vi "Set Error Line Format.vi"(8 "error in (no error)":errorcluster, 10 "Error Line Format":string, 11 "HSE_v2_Formatter in":refnum<class "HSE_v2_Formatter.lvclass">) -> (0 "error out":errorcluster, 3 "HSE_v2_Formatter out":refnum<class "HSE_v2_Formatter.lvclass">)   [LabVIEW 2016, in "hse-logger.lvlib" / "HSE_v2_Formatter.lvclass"]
uses:
  HSE_v2_Formatter.lvclass
  HSE_v2_Formatter.lvclass/HSE_v2_Formatter.ctl
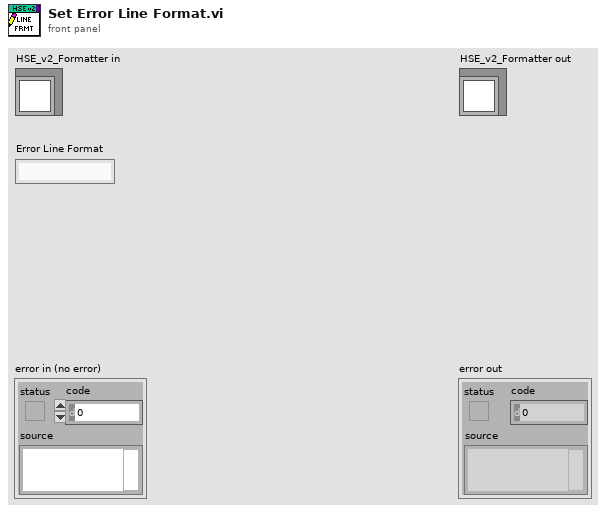
[diagram p1: front panel]
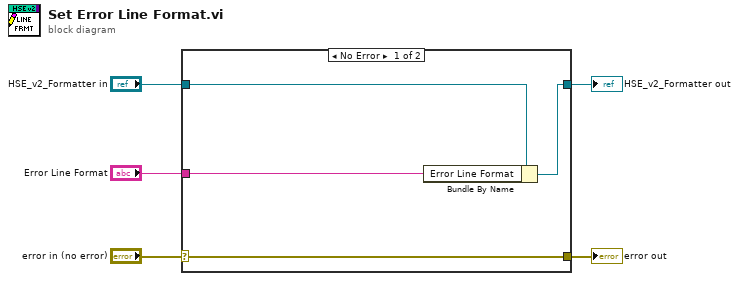
[diagram p0: block diagram]
diagram:
  n1 = case shown="No Error" "error in (no error)" {
    selector: "error in (no error)" -> [w9 w10]
    tunnel: [w9 w10] -> w4
    tunnel: [w7 w11] -> w2
    tunnel: "HSE_v2_Formatter in" -> [w8 w11]
    tunnel: "Error Line Format" -> [w6 _]
    frame No Error {
      n2 = Bundle By Name(cluster=w8, "Error Line Format"=w6) -> (w7:refnum<class "HSE_v2_Formatter.lvclass">)
    }
    frame Error {
    }
  }
  "error out" <- w4
  "HSE_v2_Formatter out" <- w2
